vi "Sand Fall Till the Void Improved.vi"(3 "Possible Movements":cdb[](array[numeric]), 4 "Sand Source Coordinates":cdb, 5 "Rock Grid":set{cdb}(c389)) -> (0 "Bounds":T1, 1 "Sand Fall steps":T2(array[cluster]), 2 "Sand Grid":set{cdb}(c389))   [LabVIEW 2020, in "AoC 2022.lvlib"]
uses:
  AoC 2022.lvlib
  f83a1fb8-6652-4940-98ed-d4d1fe9cdb95.vi
  a2426853-035e-405c-9e35-7dca2c704f70.vi
  f83a1fb8-6652-4940-98ed-d4d1fe9cdb95.vi/7c7783df-fd5a-49d9-9b7a-63cc9fb0e4e5.vi
panel:
  out "size":i32
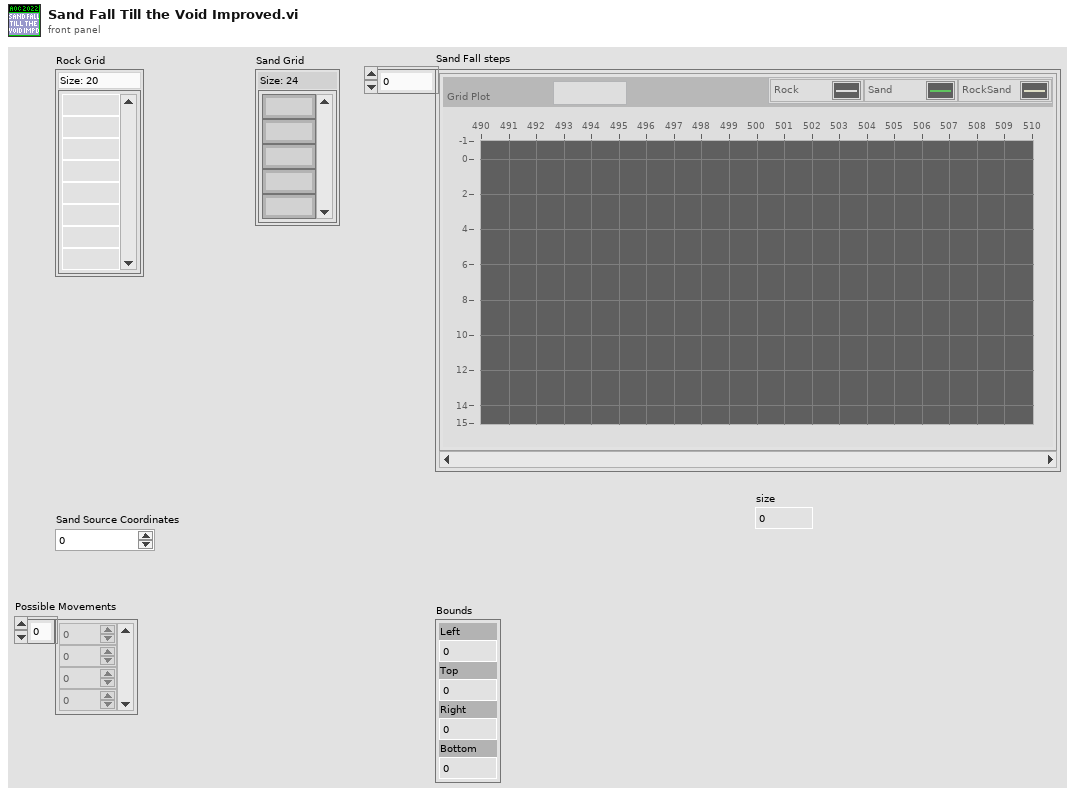
[diagram p1: front panel]
types:
  T1 = cluster{"Left":i16, "Top":i16, "Right":i16, "Bottom":i16}
  T2 = cluster{"Grid Plot":cluster{cluster{i32, i32}[]}[]}[]
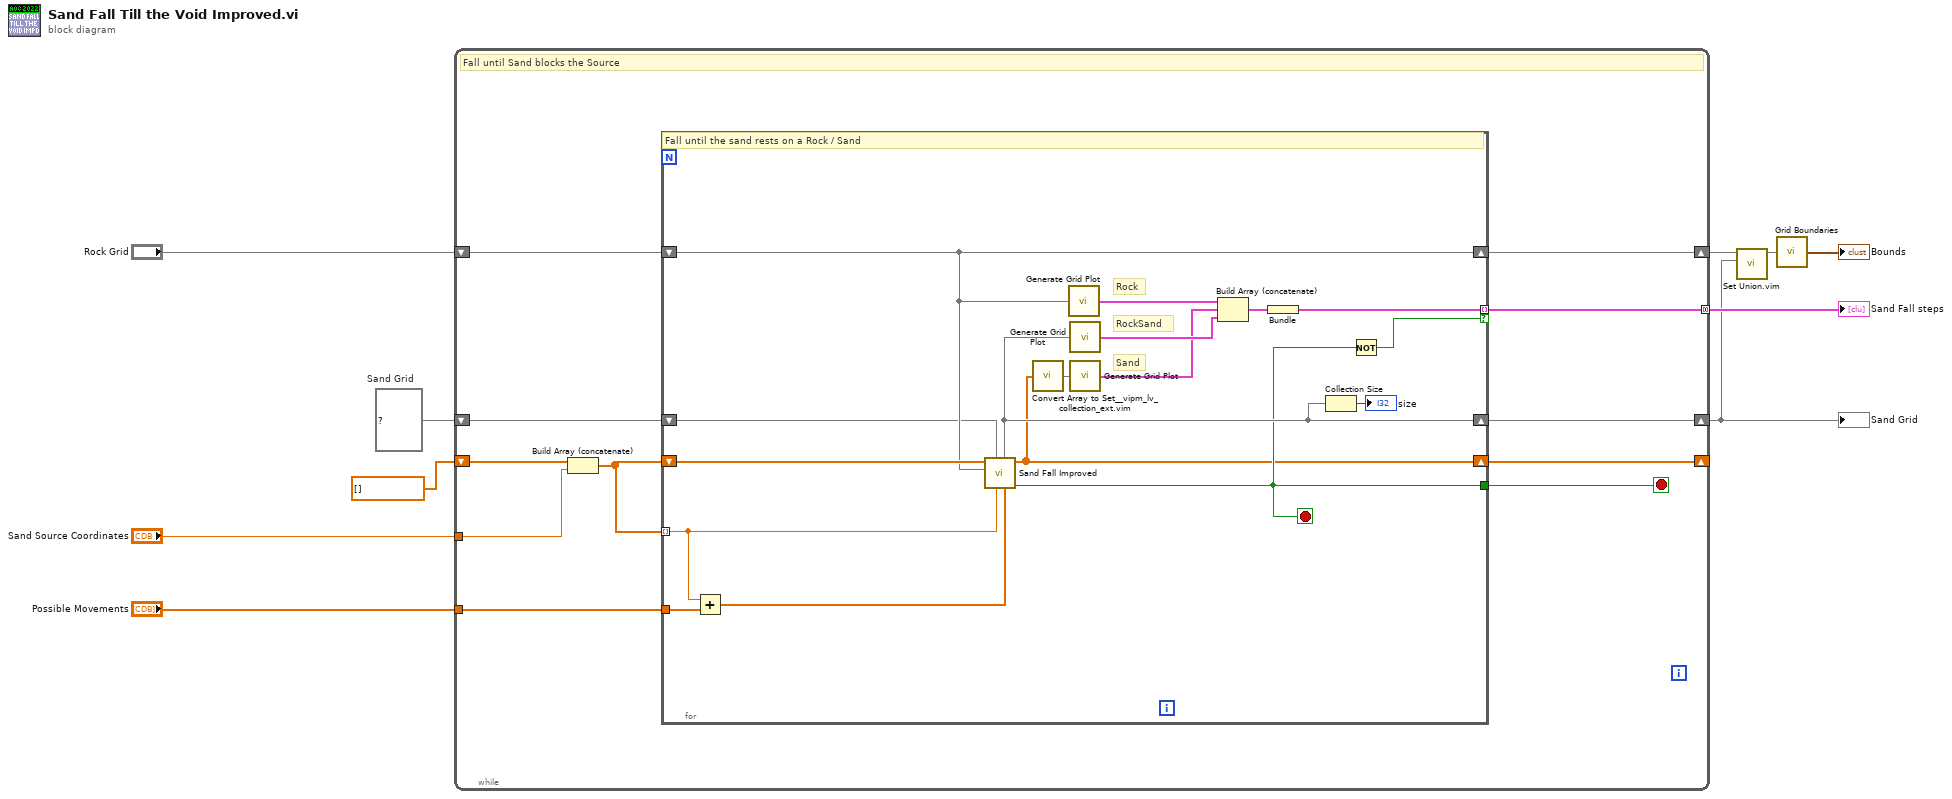
[diagram p0: block diagram]
diagram:
  w6 = set{cdb} {}  # Sand Grid
  n1 = while {
    shift-right: [w18] -> _
    shift-left: cdb[] [] ("Coordinates") -> [w15]
    tunnel: "Possible Movements" -> [w21]
    tunnel: [w19] -> w7 mode=concatenating
    shift-right: [w16] -> w3
    shift-left: "Rock Grid" -> [w17]
    tunnel: "Sand Source Coordinates" -> [w12]
    shift-right: [w14] -> w2
    shift-left: w6 -> [w13]
    stop <- w20 stop-if-true
    # "Fall until Sand blocks the Source"
    n2 = Build Array (concatenate)(w15, w12) -> (w11:cdb[])
    n3 = for {
      shift-right: [w26] -> w18
      shift-left: w11 -> [w35]
      tunnel: w21 -> [w38]
      tunnel: [w24] -> w19 mode=indexing if=w37
      shift-right: [w34] -> w16
      shift-left: w17 -> [w34]
      tunnel: w11 -> [w32] mode=indexing
      shift-right: [w28] -> w14
      shift-left: w13 -> [w31]
      tunnel: [w27] -> w20
      stop <- w27 stop-if-true
      # "RockSand"
      # "Sand"
      # "Rock"
      # "Fall until the sand rests on a Rock / Sand"
      n4 = Add(x=w32, y=w38) -> (x+y=w33:cdb[])
      n5 = call "Sand Fall Improved.vi"("Next Possible Locations"=w33, "Current Sand Location"=w32, "RockSand Grid in"=w31, "Rock Grid"=w34, "Falling Sand List in"=w35) -> ("Falling into Void ?"=w27:bool, "Falling Sand List out"=w26:cdb[], "RockSand Grid out"=w28:set{cdb})  [unwired: 4 in]
      n6 = call "Convert Array to Set__vipm_lv_collection_ext.vim"("array"=w26) -> ("set"=w25:set{cdb})  [unwired: 6 in]
      n7 = call "Generate Grid Plot.vi"("Grid"=w34) -> ("Grid Plot"=w30:cluster{cluster{i32, i32}[]}[])
      n8 = call "Generate Grid Plot.vi"("Grid"=w28) -> ("Grid Plot"=w23:cluster{cluster{i32, i32}[]}[])
      n9 = call "Generate Grid Plot.vi"("Grid"=w25) -> ("Grid Plot"=w22:cluster{cluster{i32, i32}[]}[])
      n10 = Build Array (concatenate)(w30, w22, w23) -> (w29:cluster{cluster{i32, i32}[]}[])
      n11 = Bundle(w29) -> (w24:cluster{cluster{cluster[]}[]})  [unwired: 1 in]
      n12 = Collection Size(1:w28) -> (0:→"size":i32)
      n13 = Not(x=w27) -> (.not. x?=w37:bool)
    }
  }
  "Sand Grid" <- w2
  "Sand Fall steps" <- w7
  n14 = call "Set Union.vim"("set 2"=w2, "set 1"=w3) -> ("union"=w1:set{cdb})  [unwired: 9 in]
  n15 = call "Grid Boundaries.vi"("Grid"=w1) -> ("Bounds"=→"Bounds":T1)
